vi "Insert Indicators to [4,4] Array.vi"(7 "indicators":refnum<vi>[](array[refnum]), 9 "2-D controls references":refnum<vi>[][](array[refnum]), 11 "controls":refnum<vi>[](array[refnum])) -> (1 "2-D controls references out":refnum<vi>[][](array[refnum]))   [LabVIEW 2018, in "NISAST VI Scripting.lvlib" / "VI.lvlib" / "Front Panel.lvlib"]
uses:
  Front Panel.lvlib
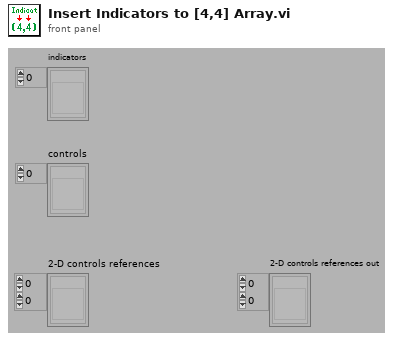
[diagram p1: front panel]
types:
  T1 = cluster{"Index (row)":i32, "Disabled Index (col)":i32}[]
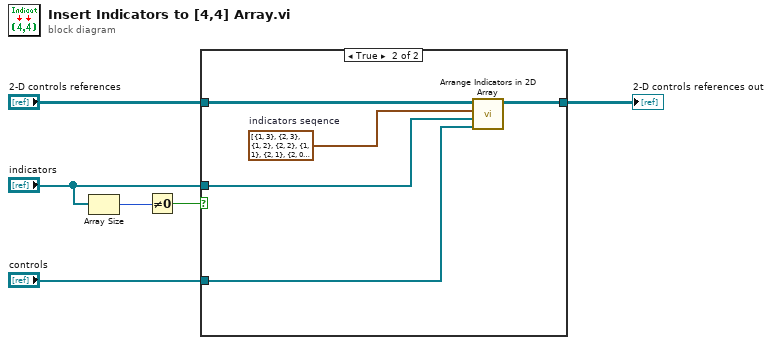
[diagram p0: block diagram]
diagram:
  n1 = Array Size(array="indicators") -> (size(s)=w1:i32)
  n2 = Not Equal To 0?(x=w1) -> (x != 0?=w4:bool)
  n3 = case shown="True" w4 {
    tunnel: "2-D controls references" -> [w7 w12]
    tunnel: [w7 w9] -> w3
    tunnel: "indicators" -> [_ w10]
    tunnel: "controls" -> [_ w11]
    frame False {
    }
    frame True {
      w8 = T1 [{"Index (row)"=1, "Disabled Index (col)"=3}, {"Index (row)"=2, "Disabled Index (col)"=3}, {"Index (row)"=1, "Disabled Index (col)"=2}, {"Index (row)"=2, "Disabled Index (col)"=2}, {"Index (row)"=1, "Disabled Index (col)"=1}, {"Index (row)"=2, "Disabled Index (col)"=1}, {"Index (row)"=2, "Disabled Index (col)"=0}, {"Index (row)"=1, "Disabled Index (col)"=0}, {"Index (row)"=0, "Disabled Index (col)"=0}]  # indicators seqence
      n4 = call "Arrange Indicators in 2D Array.vi"("controls"=w11, "indicators"=w10, "indicators seqence"=w8, "2-D references array"=w12) -> ("2-D references array out"=w9:refnum<vi>[][])  [unwired: 7 out]
    }
  }
  "2-D controls references out" <- w3
